vi "dvp Vi Set Noise Reduct2d.vi"(10 "NoiseReduct2d":i32, 11 "handle":u32) -> (3 "function return":u32(ring))   [LabVIEW 2018, in "LabViewDVPCamera.lvlib"]
doc: "LabviewDvp2Api dvpStatus dvpViSetNoiseReduct2d(dvpHandle handle, dvpInt32 NoiseReduct2d);"
uses:
  LabViewDVPCamera.lvlib
  LabViewDVPCamera/LabViewDVPCamera.dll
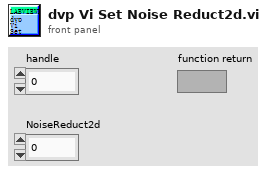
[diagram p1: front panel]
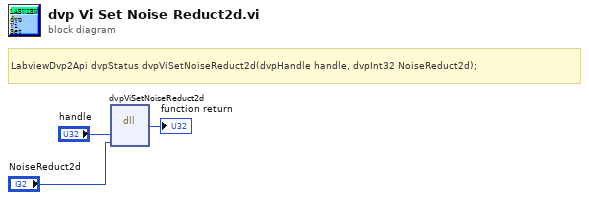
[diagram p0: block diagram]
diagram:
  # "LabviewDvp2Api dvpStatus dvpViSetNoiseReduct2d(dvpHandle handle, dvpInt32 NoiseReduct2d);"
  n1 = dll-call lib="C:/Program Files (x86)/DVP2 Labview cn 64/Sample/LabViewDVPCamera/LabViewDVPCamera.*" fn="dvpViSetNoiseReduct2d"("handle"="handle", "NoiseReduct2d"="NoiseReduct2d") -> (→"function return":u32)  [unwired: 5 in, 2 out]
